vi "Get Front Panel Object Types 2013 NIVerifed.vi"() -> ()   [LabVIEW 2016]
panel:
  in  "error in (no error)":errorcluster
  out "error out":errorcluster
  out "Front Panel Object Types":string[](array[string])
  # "Overview: This example demonstrates how to retrieve the data type of all front panel objects through the use of VI Server, Property Nodes & Scripting Property Nodes. \nRequirements: LabVIEW 2013 (or compatible)\nInstructions:\n1. Run the VI\n2. The VI will launch a file browser dialog, select the VI of your choice, or select the example front panel included in the project \"Test Front Panel.vi\"\n 3. The code will run and populate the array with the Front Panel Object Types. These can be compared to the selected VI, remembering that the array is populated based on the index of the front panel control."
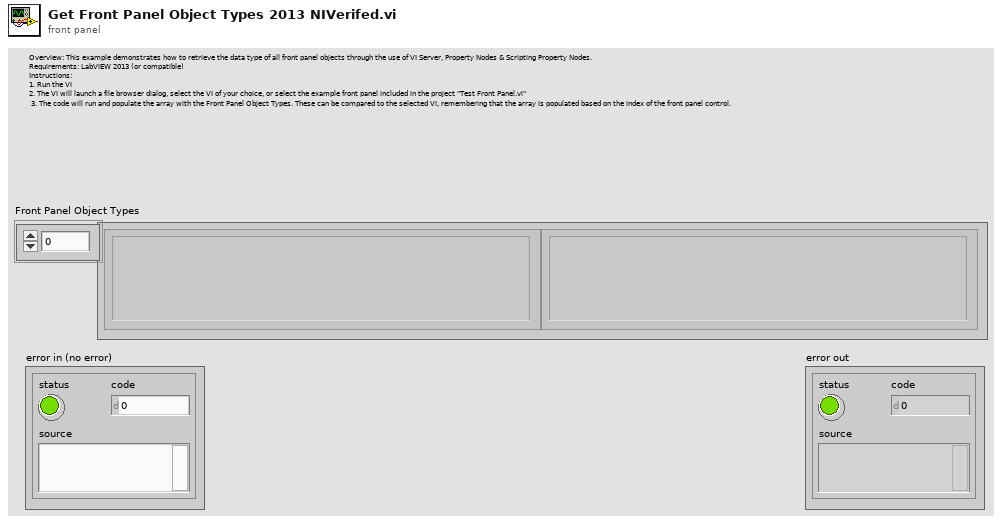
[diagram p1: front panel]
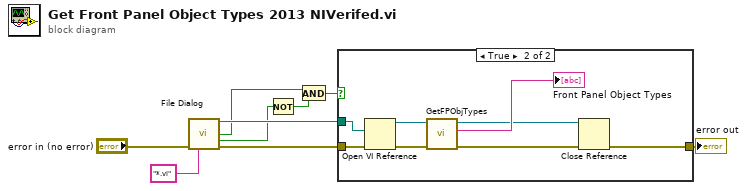
[diagram p0: block diagram]
diagram:
  n1 = call "File Dialog"("error in"="error in (no error)", "pattern (all files)"="*.vi" ("default name")) -> ("selected path"=w9:path, "exists"=w1:bool, "cancelled"=w6:bool, "error out"=w7:errorcluster)  [unwired: 10 in]
  n2 = Not(x=w6) -> (.not. x?=w3:bool)
  n3 = And(x=w1, y=w3) -> (x .and. y?=w2:bool)
  n4 = case shown="True" w2 {
    tunnel: w9 -> [_ w12]
    tunnel: w7 -> [w10 w11]
    tunnel: [w10 w13] -> w5
    frame False {
    }
    frame True {
      n5 = Open VI Reference(vi path=w12, error in (no error)=w11) -> (vi reference=w18:refnum<vi>, error out=w17:errorcluster)  [unwired: 4 in]
      n6 = call "GetFPObjTypes.vi"("error in (no error)"=w17, "Object Reference"=w18) -> ("error out"=w14:errorcluster, "Object Type"=→"Front Panel Object Types":string, "reference out"=w15:refnum<vi>)  [unwired: 7 in]
      n7 = Close Reference(reference=w15, error in (no error)=w14) -> (error out=w13:errorcluster)
    }
  }
  "error out" <- w5
